vi "add.vi"(1 "X":dbl) -> (0 "X*Y":dbl)   [LabVIEW 2015]
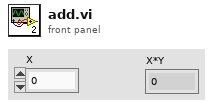
[diagram p1: front panel]
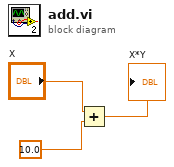
[diagram p0: block diagram]
diagram:
  n1 = Add(x="X", y=10.0) -> (x+y=→"X*Y":dbl)
